vi "PrepareMeasurementSettings.vi"(8 "error in (no error)":errorcluster, 10 "MeasConfigType":T1, 11 "Avantes in":refnum<class "Avantes.lvclass">) -> (0 "error out":errorcluster, 3 "Avantes out":refnum<class "Avantes.lvclass">)   [LabVIEW 2020, in "Avantes.lvclass"]
uses:
  <instrlib>/Classes/CCD/Avantes/Avantes.lvclass
  <instrlib>/Classes/CCD/Avantes/MeasConfigType.ctl
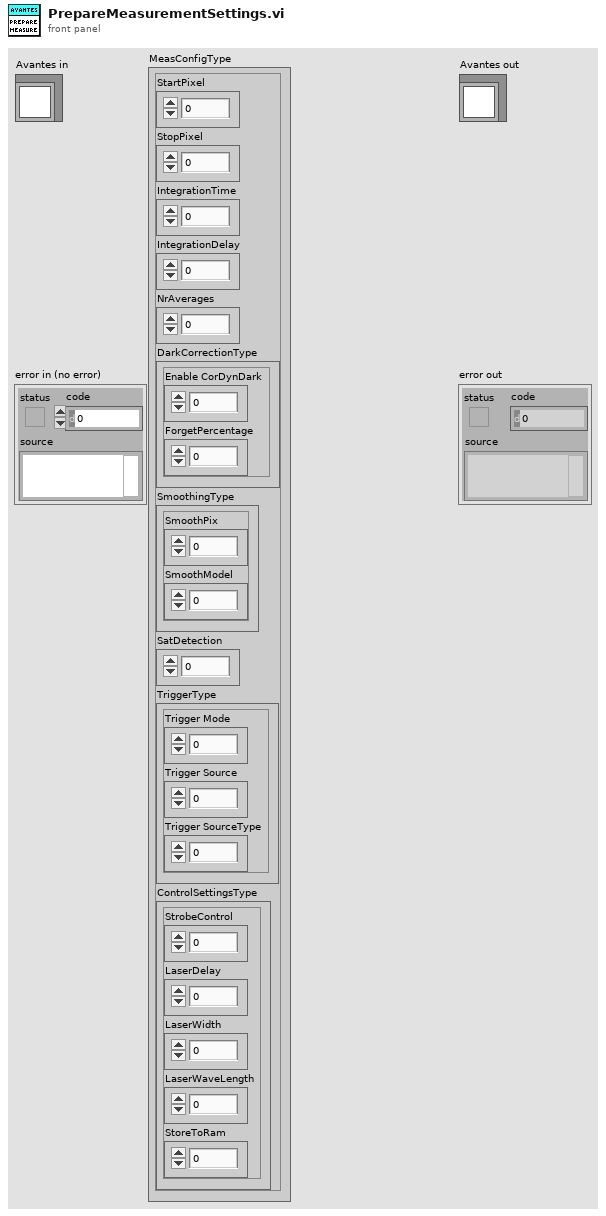
[diagram p1: front panel]
types:
  T1 = typedef "Avantes.lvclass/MeasConfigType.ctl" = cluster{"StartPixel":u16, "StopPixel":u16, "IntegrationTime":sgl, "IntegrationDelay":u32, "NrAverages":u32, "DarkCorrectionType":cluster{"Enable CorDynDark":u8, "ForgetPercentage":u8}, "SmoothingType":cluster{"SmoothPix":u16, "SmoothModel":u8}, "SatDetection":u8, "TriggerType":cluster{"Trigger Mode":u8, "Trigger Source":u8, "Trigger SourceType":u8}, "ControlSettingsType":cluster{"StrobeControl":u16, "LaserDelay":u32, "LaserWidth":u32, "LaserWaveLength":sgl, "StoreToRam":u16}}
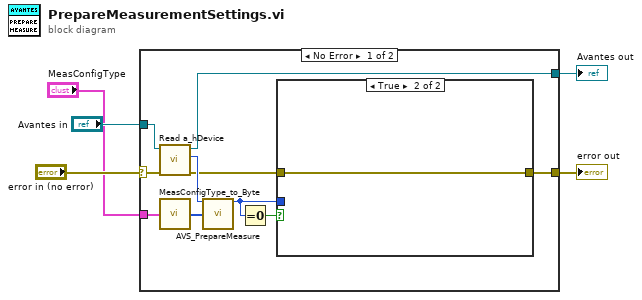
[diagram p0: block diagram]
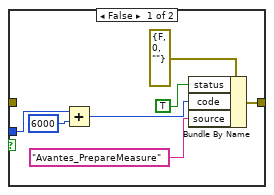
[diagram p2: hidden frame]
diagram:
  n1 = case shown="No Error" "error in (no error)" {
    selector: "error in (no error)" -> [w13 w25]
    tunnel: [w7 w25] -> w4
    tunnel: [w10 w24] -> w2
    tunnel: "Avantes in" -> [w14 w24]
    tunnel: "MeasConfigType" -> [w15 _]
    frame No Error {
      n2 = call-dynamic "Read a_hDevice.vi"("error in (no error)"=w13, "Avantes in"=w14) -> ("error out"=w8:errorcluster, "a_hDevice"=w12:i32, "Avantes out"=w10:refnum<class "Avantes.lvclass">)  [unwired: 7 in]
      n3 = call <instrlib>:"MeasConfigType_to_Byte.vi"("MeasConfigType"=w15) -> ("Byte Array"=w11:u8[])  [unwired: 4 in]
      n4 = call <instrlib>:"AVS_PrepareMeasure.vi"("a_hDevice"=w12, "MeasConfArray"=w11) -> ("Output Value"=w6:i32)  [unwired: 13 in]
      n5 = Equal To 0?(x=w6) -> (x = 0?=w9:bool)
      n6 = case shown="True" w9 {
        tunnel: w8 -> [_ w23]
        tunnel: [w16 w23] -> w7
        tunnel: w6 -> [w20 _]
        frame False {
          n7 = Add(x=w20, y=6000) -> (x+y=w18:i32)
          n8 = Bundle By Name(cluster=errorcluster {"status"=FALSE, "code"=0, "source"=""} ("error constant"), "status"=TRUE, "code"=w18, "source"="Avantes_PrepareMeasure") -> (w16:errorcluster)
        }
        frame True {
        }
      }
    }
    frame Error {
    }
  }
  "error out" <- w4
  "Avantes out" <- w2
